vi "Contour_ToVolts.vi"(10 "N Contour Points":i32, 11 "Array In":cluster{"x":sgl, "y":sgl}[](array[cluster])) -> (2 "Y Array Out":dbl[](array[numeric]), 3 "X Array Out":dbl[](array[numeric]))   [LabVIEW 2015]
panel:
  out "Left":i16
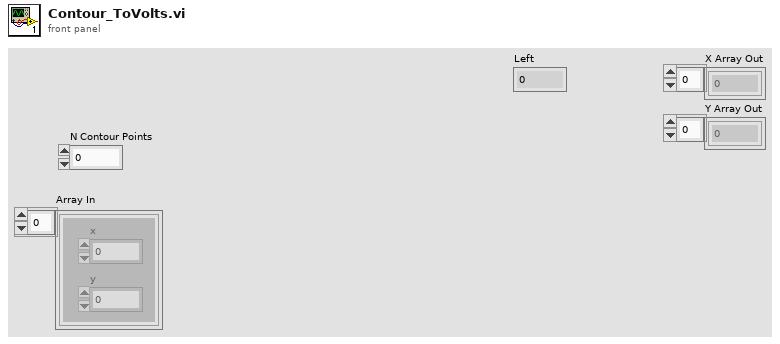
[diagram p1: front panel]
types:
  T1 = typedef "LVRectTypeDef.ctl" = cluster{"Left":i16, "Top":i16, "Right":i16, "Bottom":i16}
  T2 = cluster{"Xpixels":i32, "Vxminref":dbl, "Vxmaxref":dbl, "P":dbl, "Ypixels":i32, "Vyminref":dbl, "Vymaxref":dbl, "srate":sgl, "sAOxy":i32, "timeout":dbl, "type":string, "date":string, "time":string, "Colormap":u16, "Drawing Mode":u16, "Scanning Mode":u16, "square pixels":bool, "square matrix":bool, "Xpixels Img":i32, "Vx-min Img":dbl, "VX-max Img":dbl, "Ypixels Img":i32, "Vy-min Img":dbl, "Vy-max Img ":dbl, "Angle Img":dbl, "autoshutter":bool, "finite":bool, "cont":bool, "wavdet":bool, "measpoints":i32, "avpp":i32, "bufferAO":i32, "bufferAI":i32, "starttick":u32, "waveform":path, "Vx-ref":dbl, "Vy-ref":dbl, "refreshrate":dbl, "refreshbuffer":i32, "tt_cycles":i32, "motorref":refnum<k7>, "mirrorswitch":refnum<k7>, "sample mode":i32, "maxbufferAI":i32, "srateAODO":sgl, "bin":sgl, "Pel":sgl, "Angle draw":dbl, "srate Img":sgl, "ROIimg_plotbounds":T1, "auto OD":bool, "ODfilt":u16, "aAI":i32[], "aCI":i32[], "aAO":u32[], "aDO":u32[], "refwfsize":dbl, "Lifetime":bool, "Vz-Img":dbl, "Vz-ref":dbl, "Vz-reset":dbl, "AIoverride":bool, "aAS":u32[], "XYZstart":dbl[]}
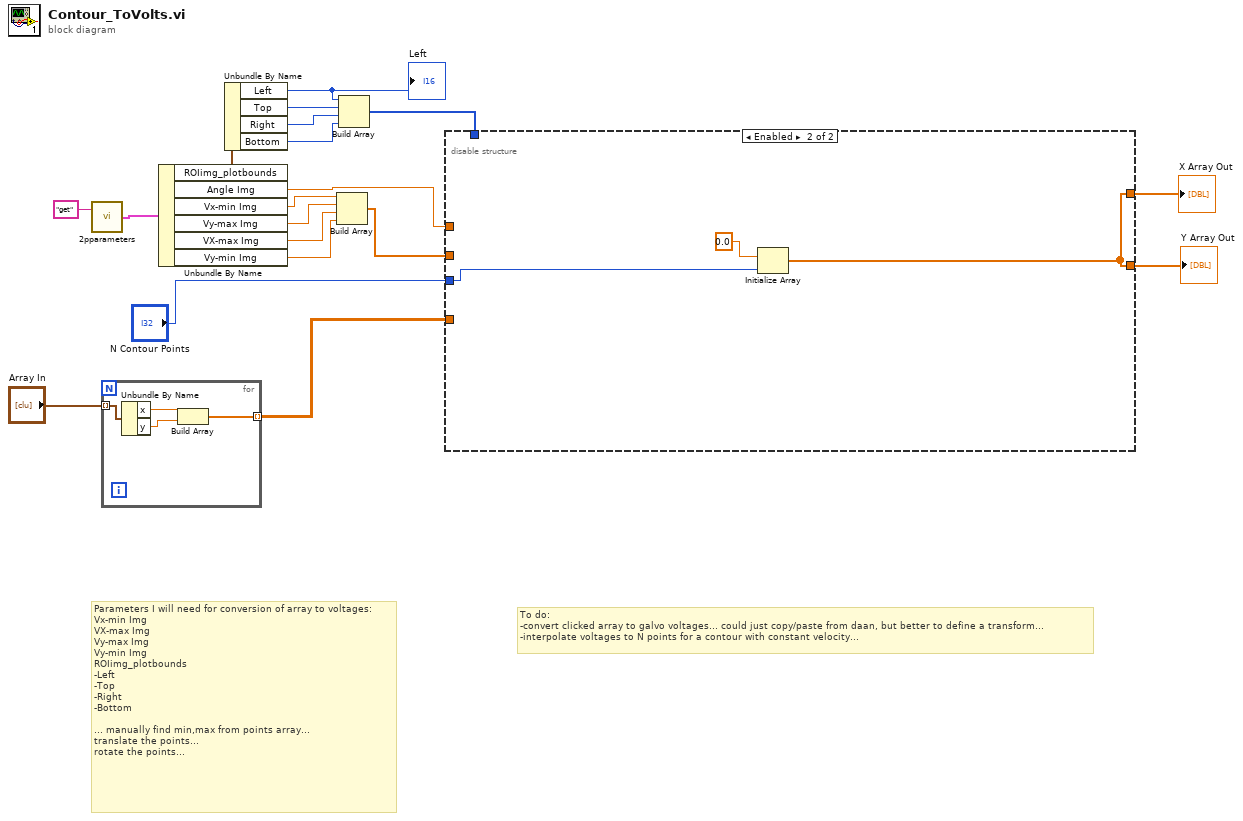
[diagram p0: block diagram]
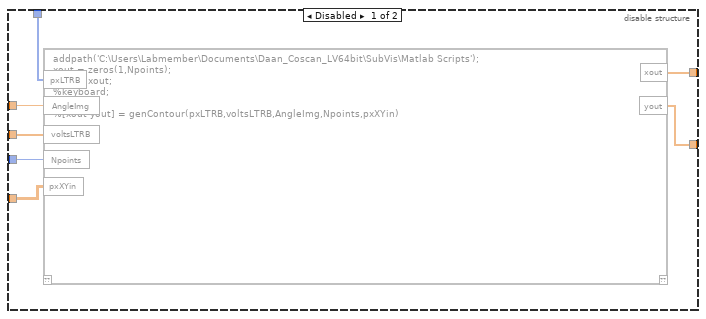
[diagram p2: hidden frame]
diagram:
  # "To do:\n-convert clicked array to galvo voltages... could just copy/paste from daan, but better to define a transform...\n-interpolate voltages to N points for a contour with constant velocity..."
  # "Parameters I will need for conversion of array to voltages:\nVx-min Img\nVX-max Img\nVy-max Img\nVy-min Img\nROIimg_plotbounds\n-Left\n-Top\n-Right\n-Bottom\n\n... manually find min,max from points array...\ntranslate the points...\nrotate the points..."
  n1 = call "2pparameters.vi"("command"="get") -> ("params out"=w19:T2)  [unwired: 1 in]
  n2 = for {
    tunnel: "Array In" -> [w23] mode=indexing
    tunnel: [w20] -> w3 mode=indexing
    n3 = Unbundle By Name(w23) -> ("x"=w22:sgl, "y"=w21:sgl)
    n4 = Build Array(w22, w21) -> (w20:sgl[])
  }
  n5 = Unbundle By Name(w19) -> ("ROIimg_plotbounds"=w17:T1, "Angle Img"=w6:dbl, "Vx-min Img"=w11:dbl, "Vy-max Img"=w10:dbl, "VX-max Img"=w9:dbl, "Vy-min Img"=w8:dbl)
  n6 = Unbundle By Name(w17) -> ("Left"=w13:i16, "Top"=w14:i16, "Right"=w15:i16, "Bottom"=w16:i16)
  "Left" <- w13
  n7 = Build Array(w11, w10, w9, w8) -> (w7:dbl[])
  n8 = Build Array(w13, w14, w15, w16) -> (w12:i16[])
  n9 = disable-structure shown="Enabled" {
    disable-tunnel: w12 -> [w30 _]
    disable-tunnel: w7 -> [w29 _]
    disable-tunnel: w6 -> [w28 _]
    disable-tunnel: "N Contour Points" -> [w27 w32]
    disable-tunnel: w3 -> [w26 _]
    disable-tunnel: [w25 w31] -> w2
    disable-tunnel: [w24 w31] -> w1
    frame Disabled {
      n10 = script code="addpath('C:\\Users\\Labmember\\Documents\\Daan_Coscan_LV64bit\\SubVis\\Matlab Scripts');\nxout = zeros(1,Npoints);\nyout = xout;\n%keyboard;\n\n%[xout yout] = genContour(pxLTRB,voltsLTRB,AngleImg,Npoints,pxXYin)"("pxLTRB"=w30, "voltsLTRB"=w29, "AngleImg"=w28, "Npoints"=w27, "pxXYin"=w26) -> ("xout"=w25:dbl[], "yout"=w24:dbl[])  [unwired: 1 in, 1 out]
    }
    frame Enabled {
      n11 = Initialize Array(0.0 ("P"), w32) -> (w31:dbl[])
    }
  }
  "X Array Out" <- w2
  "Y Array Out" <- w1
